vi "Read estimated array size.vi"(8 "error in":errorcluster, 11 "TEC configuration in":refnum<class "TEC configuration.lvclass">) -> (0 "error out":errorcluster, 2 "estimated array size":u16, 3 "TEC configuration out":refnum<class "TEC configuration.lvclass">)   [LabVIEW 2013, in "TEC configuration.lvclass"]
uses:
  TEC configuration.lvclass
  TEC configuration.lvclass/TEC configuration.ctl
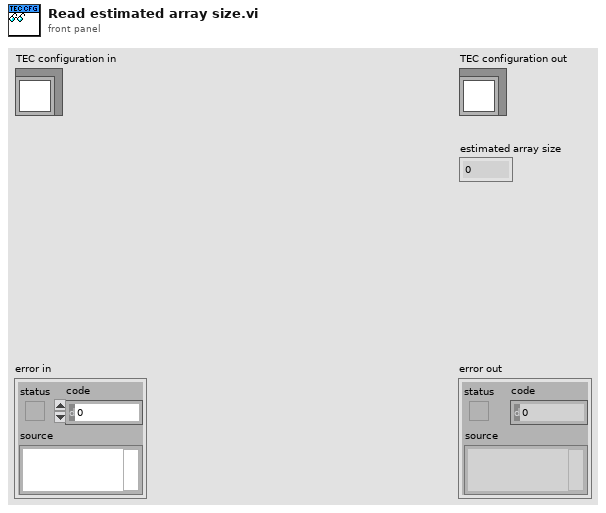
[diagram p1: front panel]
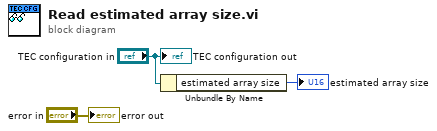
[diagram p0: block diagram]
diagram:
  n1 = Unbundle By Name("TEC configuration in") -> ("estimated array size"=→"estimated array size":u16)
  "error out" <- "error in"
  "TEC configuration out" <- "TEC configuration in"
